vi "Init Dialog_TwoButtons.vi"(4 "Button #2 text (Cancel)":string="Cancel", 5 "Allow to close? (T)":bool=TRUE, 6 "Button #1 text (OK)":string="OK", 7 "Dialog_2Buttons in":refnum<class "Dialog_TwoButtons.lvclass">, 8 "error in (no error)":errorcluster, 9 "Timeout (-1)":i32=-1, 10 "Message":string, 11 "Dialog Title":string) -> (0 "error out":errorcluster, 3 "Dialog_2Buttons out":refnum<class "Dialog_TwoButtons.lvclass">)   [LabVIEW 2012, in "Dialog_TwoButtons.lvlib" / "Dialog_TwoButtons.lvclass"]
doc: "Initialization VI for a 2-button dialog box."
uses:
  Dialog_TwoButtons.lvclass
  Dialog_TwoButtons.lvclass/Dialog_TwoButtons.ctl
  Dialog/Dialog/Dialog.lvclass
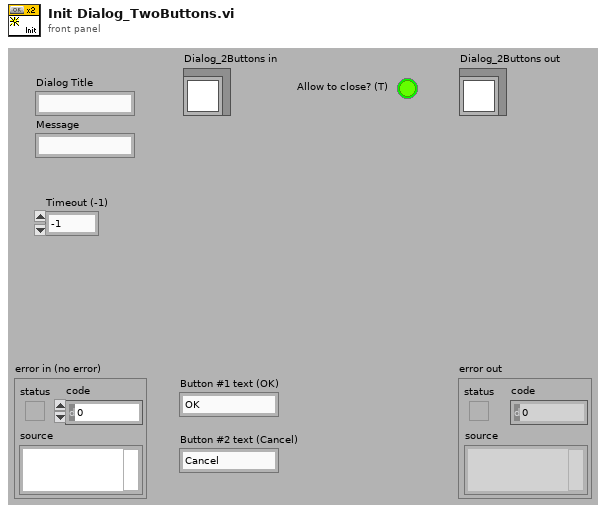
[diagram p1: front panel]
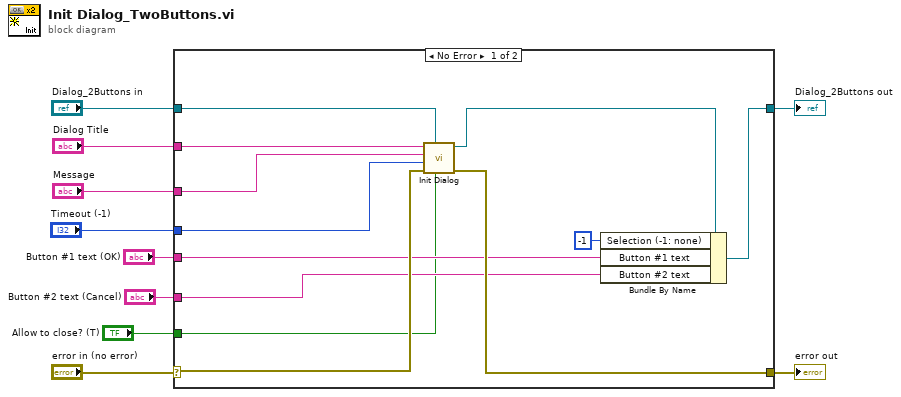
[diagram p0: block diagram]
diagram:
  n1 = case shown="No Error" "error in (no error)" {
    selector: "error in (no error)" -> [w20 w24]
    tunnel: [w21 w24] -> w9
    tunnel: [w15 w23] -> w7
    tunnel: "Dialog_2Buttons in" -> [w22 w23]
    tunnel: "Dialog Title" -> [w19 _]
    tunnel: "Message" -> [w18 _]
    tunnel: "Button #1 text (OK)" -> [w14 _]
    tunnel: "Button #2 text (Cancel)" -> [w13 _]
    tunnel: "Timeout (-1)" -> [w12 _]
    tunnel: "Allow to close? (T)" -> [w11 _]
    frame No Error {
      n2 = call "Init Dialog.vi"("Allow to close? (T)"=w11, "Dialog in"=w22, "error in (no error)"=w20, "Timeout (-1)"=w12, "Message"=w18, "Dialog Title"=w19) -> ("error out"=w21:errorcluster, "Dialog out"=w16:refnum<class "Dialog_TwoButtons.lvclass">)  [unwired: 4 out]
      n3 = Bundle By Name(cluster=w16, "Selection (-1: none)"=i8 -1, "Button #1 text"=w14, "Button #2 text"=w13) -> (w15:refnum<class "Dialog_TwoButtons.lvclass">)
    }
    frame Error {
    }
  }
  "error out" <- w9
  "Dialog_2Buttons out" <- w7
